vi "Mouse Up.vi"(7 "Map Model in":refnum<class "Map Model.lvclass">, 8 "error in (no error)":errorcluster, 10 "Position":T1, 11 "Pan in":refnum<class "Pan.lvclass">) -> (0 "error out":errorcluster, 3 "Pan out":refnum<class "Pan.lvclass">, 5 "Map Model out":refnum<class "Map Model.lvclass">)   [LabVIEW 2020, in "Map Model.lvlib" / "Pan.lvclass"]
uses:
  Pan.lvclass
  E:/Project/Labview-Projects/Completed projects/Map Editor/Models/Map Model/Tools/Tool/Tool.lvclass
  <vilib>/Utility/miscctls.llb/LVPoint32TypeDef.ctl
  Map Model/Map Model.lvclass
  Tool/Tool.lvclass/Tool.ctl
  Map Model/Map Model.lvclass/Map Model.ctl
  Undoable Tool/Undoable Tool.lvclass
  Tool/Tool.lvclass
panel:
  # "NOTICE -- YOU MUST LEAVE THIS NOTICE IN PLACE.\n\nCopyright (c) 2017, LIANG LIU Shawn.Liu.cn@gmail.com\nAll rights reserved.\n\nRedistribution and use in source and binary forms, with or without modification, are permitted provided that the following conditions are met:\n-Redistributions of source code must retain the above copyright notice, this list of conditions and the following disclaimer.\n-Redistributions in binary form must reproduce the above copyright notice, this list of conditions and the following disclaimer in the documentation and/or other materials provided with the distribution.\n-Neither the name of the eLp nor the names of its contributors may be used to endorse or promote products derived from this software without specific prior written permission.\n\nTHIS SOFTWARE IS PROVIDED BY THE COPYRIGHT HOLDERS AND CONTRIBUTORS \"AS IS\" AND ANY EXPRESS OR IMPLIED WARRANTIES, INCLUDING, BUT NOT LIMITED TO, THE IMPLIED WARRANTIES OF MERCHANTABILITY AND FITNESS FOR A PARTICULAR PURPOSE ARE DISCLAIMED. IN NO EVENT SHALL THE COPYRIGHT HOLDER OR CONTRIBUTORS BE LIABLE FOR ANY DIRECT, INDIRECT, INCIDENTAL, SPECIAL, EXEMPLARY, OR CONSEQUENTIAL DAMAGES (INCLUDING, BUT NOT LIMITED TO, PROCUREMENT OF SUBSTITUTE GOODS OR SERVICES; LOSS OF USE, DATA, OR PROFITS; OR BUSINESS INTERRUPTION) HOWEVER CAUSED AND ON ANY THEORY OF LIABILITY, WHETHER IN CONTRACT, STRICT LIABILITY, OR TORT (INCLUDING NEGLIGENCE OR OTHERWISE) ARISING IN ANY WAY OUT OF THE USE OF THIS SOFTWARE, EVEN IF ADVISED OF THE POSSIBILITY OF SUCH DAMAGE."
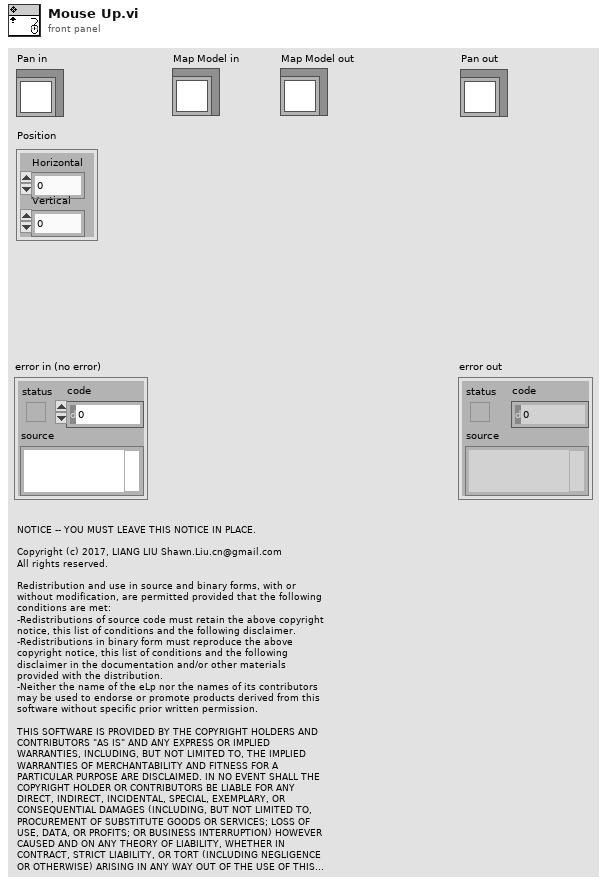
[diagram p1: front panel]
types:
  T1 = typedef "LVPoint32TypeDef.ctl" = cluster{"Horizontal":i32, "Vertical":i32}
  T2 = typedef "LVPointTypeDef.ctl" = cluster{"Horizontal":i16, "Vertical":i16}
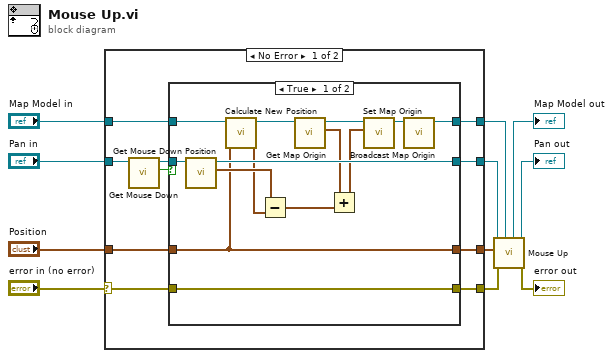
[diagram p0: block diagram]
diagram:
  n1 = case shown="No Error" "error in (no error)" {
    selector: "error in (no error)" -> [w17 w43]
    tunnel: "Map Model in" -> [w21 w42]
    tunnel: "Pan in" -> [w20 w41]
    tunnel: [w19 w40] -> w8
    tunnel: "Position" -> [w18 w40]
    tunnel: [w16 w42] -> w5
    tunnel: [w15 w41] -> w4
    tunnel: [w14 w43] -> w3
    frame No Error {
      n2 = call "Get Mouse Down.vi"("Tool in"=w20) -> ("Mouse Down"=w12:bool, "Tool out"=w13:refnum<class "Pan.lvclass">)  [unwired: 9 in]
      n3 = case shown="True" w12 {
        tunnel: w13 -> [w33 w39]
        tunnel: w21 -> [w34 w37]
        tunnel: [w30 w37] -> w16
        tunnel: [w32 w39] -> w15
        tunnel: w18 -> [w24 w36]
        tunnel: [w24 w36] -> w19
        tunnel: w17 -> [w35 w38]
        tunnel: [w35 w38] -> w14
        frame True {
          n4 = call "Get Mouse Down Position.vi"("Tool in"=w33) -> ("Mouse Down Position"=w31:T1, "Tool out"=w32:refnum<class "Pan.lvclass">)  [unwired: 9 in]
          n5 = call "Calculate New Position.vi"("Position in"=w24, "Map Model in"=w34) -> ("Position out"=w23:T1, "Map Model out"=w25:refnum<class "Map Model.lvclass">)  [unwired: 8 in]
          n6 = Subtract(x=w31, y=w23) -> (x-y=w26:T1)
          n7 = call "Get Map Origin.vi"("Map Model in"=w25) -> ("Map Origin"=w27:T2, "Map Model out"=w29:refnum<class "Map Model.lvclass">)  [unwired: 9 in]
          n8 = Add(x=w27, y=w26) -> (x+y=w22:T1)
          n9 = call "Set Map Origin.vi"("Map Origin"=w22, "Map Model in"=w29) -> ("Map Model out"=w28:refnum<class "Map Model.lvclass">)  [unwired: 9 in]
          n10 = call "Broadcast Map Origin.vi"("Map Model in"=w28) -> ("Map Model out"=w30:refnum<class "Map Model.lvclass">)  [unwired: 9 in, 1 out]
        }
        frame False {
        }
      }
    }
    frame Error {
    }
  }
  n11 = call-parent "Mouse Up.vi"("Map Model in"=w5, "error in (no error)"=w3, "Position"=w8, "Undoable Tool in"=w4) -> ("error out"=→"error out":errorcluster, "Undoable Tool out"=→"Pan out":refnum<class "Pan.lvclass">, "Map Model out"=→"Map Model out":refnum<class "Map Model.lvclass">)  [unwired: 5 in]
